vi "TargetAssist.vi"(11 "Detected Targets":T1(array[cluster]) {"Normalized Rect"."Numeric 5" format="%#_2g"; "Normalized Rect"."Numeric 3" format="%#_2g"; "Normalized Rect"."Numeric 2" format="%#_2g"; "Normalized Rect"."Numeric" format="%#_2g"}) -> (0 "Down":bool, 1 "Righ":bool, 2 "Up":bool, 3 "Left":bool, 4 "Shoot":bool)   [LabVIEW 2015]
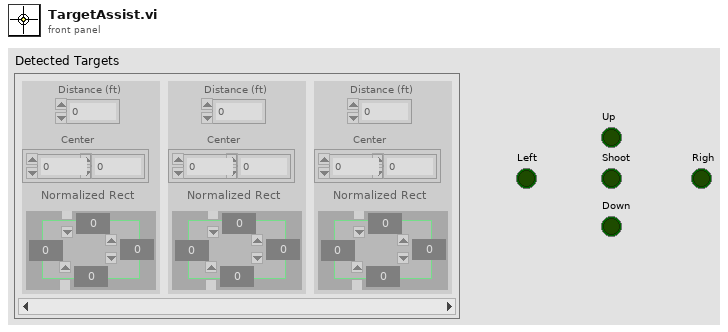
[diagram p1: front panel]
types:
  T1 = cluster{"Distance (ft)":dbl, "Center":cluster{dbl, dbl}, "Normalized Rect":cluster{"Numeric":dbl, "Numeric 2":dbl, "Numeric 3":dbl, "Numeric 5":dbl}}[]
  T2 = cluster{"Distance (ft)":dbl, "Center":cluster{dbl, dbl}, "Normalized Rect":cluster{"Numeric":dbl, "Numeric 2":dbl, "Numeric 3":dbl, "Numeric 5":dbl}}
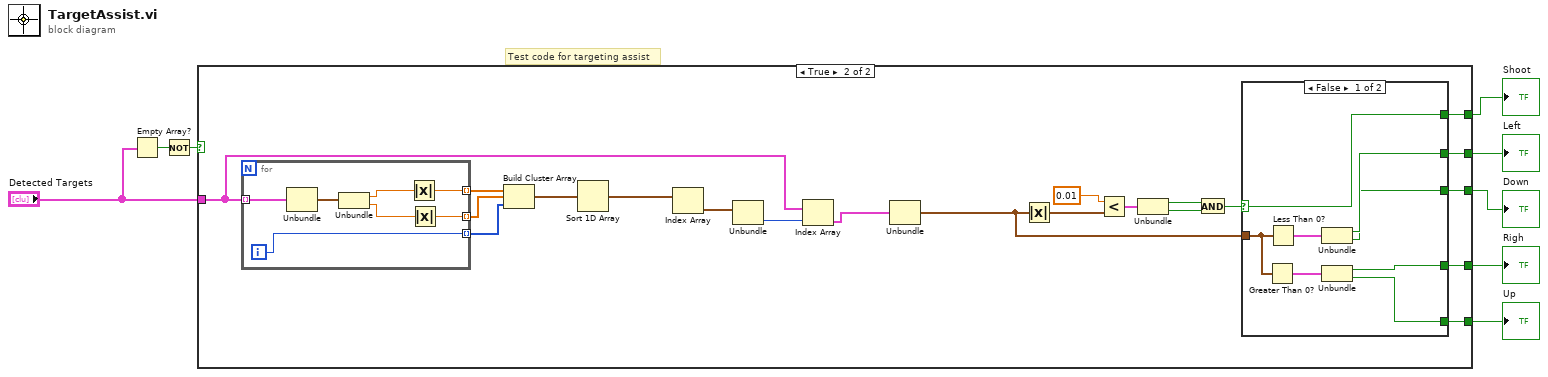
[diagram p0: block diagram]
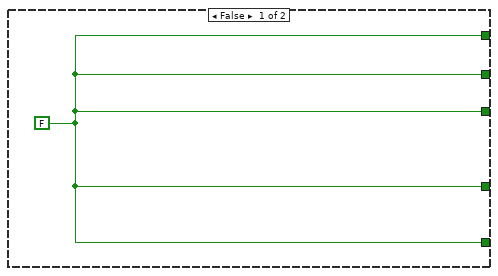
[diagram p2: hidden frame]
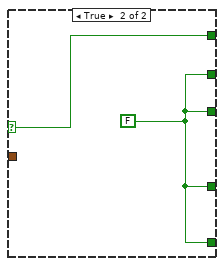
[diagram p3: hidden frame]
diagram:
  # "Test code for targeting assist"
  n1 = Empty Array?(array="Detected Targets") -> (empty?=w3:bool)
  n2 = Not(x=w3) -> (.not. x?=w2:bool)
  n3 = case shown="True" w2 {
    tunnel: "Detected Targets" -> [_ w16]
    tunnel: [w9 w28] -> w5
    tunnel: [w9 w27] -> w6
    tunnel: [w9 w26] -> w7
    tunnel: [w9 w25] -> w8
    tunnel: [w9 w23] -> w4
    frame False {
      w9 = FALSE
    }
    frame True {
      n4 = for {
        tunnel: w16 -> [w37] mode=indexing
        tunnel: [w33] -> w21 mode=indexing
        tunnel: [w32] -> w22 mode=indexing
        tunnel: [w31] -> w18 mode=indexing
        i -> [w31]
        n5 = Unbundle(w37) -> ("Center"=w36:cluster{dbl, dbl})  [unwired: 2 out]
        n6 = Unbundle(w36) -> (w35:dbl, w34:dbl)
        n7 = Absolute Value(x=w35) -> (abs(x)=w32:dbl)
        n8 = Absolute Value(x=w34) -> (abs(x)=w33:dbl)
      }
      n9 = Build Cluster Array(w22, w21, w18) -> (w20:cluster{dbl, dbl, i32}[])
      n10 = Sort 1D Array(array=w20) -> (sorted array=w19:cluster{dbl, dbl, i32}[])
      n11 = Index Array(array=w19) -> (element=w17:cluster{dbl, dbl, i32})  [unwired: 1 in]
      n12 = Unbundle(w17) -> (w15:i32)  [unwired: 2 out]
      n13 = Index Array(array=w16, index=w15) -> (element=w14:T2)
      n14 = Unbundle(w14) -> ("Center"=w13:cluster{dbl, dbl})  [unwired: 2 out]
      n15 = Absolute Value(x=w13) -> (abs(x)=w12:cluster{dbl, dbl})
      n16 = Less?(x=0.01, y=w12) -> (x < y?=w11:cluster{bool, bool})
      n17 = Unbundle(w11) -> (w30:bool, w29:bool)
      n18 = And(x=w30, y=w29) -> (x .and. y?=w24:bool)
      n19 = case shown="False" w24 {
        selector: w24 -> [w44 w47]
        tunnel: w13 -> [w43 _]
        tunnel: [w41 w46] -> w27
        tunnel: [w40 w46] -> w28
        tunnel: [w38 w46] -> w26
        tunnel: [w39 w46] -> w25
        tunnel: [w44 w47] -> w23
        frame False {
          n20 = Greater Than 0?(x=w43) -> (x > 0?=w42:cluster{bool, bool})
          n21 = Less Than 0?(x=w43) -> (x < 0?=w45:cluster{bool, bool})
          n22 = Unbundle(w45) -> (w41:bool, w39:bool)
          n23 = Unbundle(w42) -> (w40:bool, w38:bool)
        }
        frame True {
          w46 = FALSE
        }
      }
    }
  }
  "Shoot" <- w4
  "Left" <- w6
  "Righ" <- w5
  "Down" <- w8
  "Up" <- w7
